vi "sub_ntrip-client-connection-command.vi"(7 "cmd":enum16{"Get ref", "Get rtcm"}(ring), 11 "Current Ntrip account":T1={"address"="gnss.eseoul.go.kr", "port "=2101, "id"="seoul", "pwd"="seoul", "ref pt"="YONS-RTCM32-M5"}) -> (3 "hex":string)   [LabVIEW 2019]
uses:
  Ctrl/Ntrip_Account_db.ctl
panel:
  in  "ascii 2":string="GET / HTTP/1.0\r\nUser-Agent: NTRIP u-blox\r\nAccept: */*\r\nAuthorization: Basic c2VvdWw6c2VvdWw=\r\nConnection: close\r\n\r\n"
  out "ascii":string
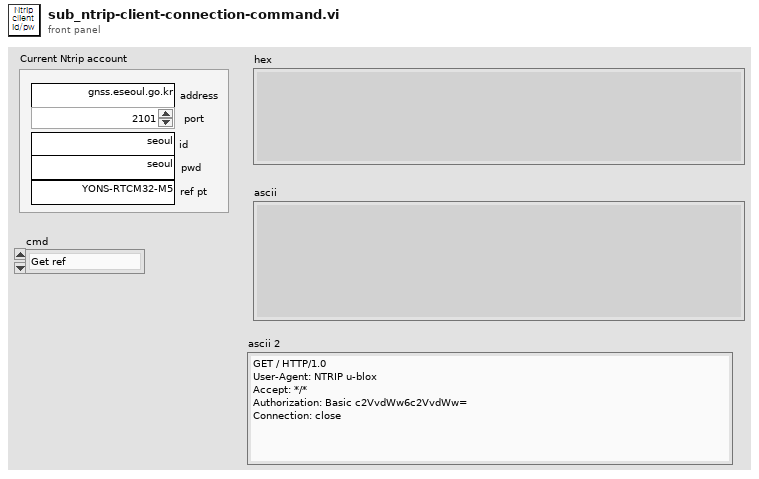
[diagram p1: front panel]
types:
  T1 = typedef "Ntrip_Account_db.ctl" = cluster{"address":string, "port ":u16, "id":string, "pwd":string, "ref pt":string}
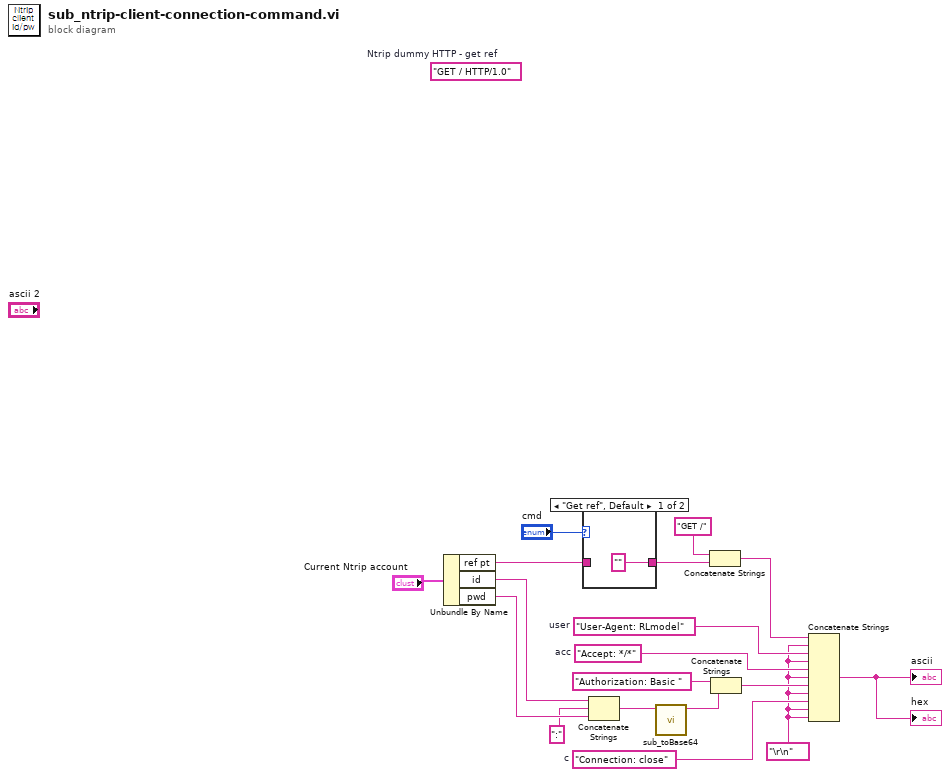
[diagram p0: block diagram]
diagram:
  w10 = "Accept: */*"  # acc
  w11 = "User-Agent: RLmodel"  # user
  w6 = "\r\n" ("string")
  w7 = "Connection: close"  # c
  (unwired) "GET / HTTP/1.0"  # Ntrip dummy HTTP - get ref
  n1 = Unbundle By Name("Current Ntrip account") -> ("ref pt"=w13:string, "id"=w17:string, "pwd"=w18:string)
  n2 = case shown="\"Get ref\", Default" "cmd" {
    tunnel: w13 -> [_ w20]
    tunnel: ["" ("문자열") w20] -> w3
    frame "Get ref", Default {
    }
    frame "Get rtcm" {
    }
  }
  n3 = Concatenate Strings(w17, ":" ("string"), w18) -> (w16:string)
  n4 = call "sub_toBase64.vi"("str-in"=w16) -> ("Base64"=w5:string)  [unwired: 10 in]
  n5 = Concatenate Strings("GET /" ("data in"), w3) -> (w2:string)
  n6 = Concatenate Strings("Authorization: Basic " ("string"), w5) -> (w8:string)
  n7 = Concatenate Strings(w2, w6, w11, w6, w10, w6, w8, w6, w7, w6, w6) -> (→"hex" →"ascii":string)
